vi "Autogenerate_Topology_Relation.vi"(5 "Goal District":string, 7 "Start District":string, 9 "PicAjust":T1={"TranslationVector"=[], "scale"=1.0, "Pitch（x) "=0.0, "Yaw（y)"=0.0, "Roll（z) "=0.0}, 10 "Cluster of 7 Type Data":T3(array[cluster])) -> (0 "District Name Array":string[](array[string]), 1 "Path Coodinate Array":dbl[][](array[numeric]), 2 "Path Relation topology":dbl[][](array[numeric]), 3 "Topology Matrix":dbl[][](array[numeric]), 4 "All Path Array":string[](array[string]), 8 "yidong":dbl[](array[numeric]))   [LabVIEW 2014]
doc: "通过数据生成各个房间、过道、楼梯的空间拓扑矩阵"
uses:
  <vilib>/Analysis/Matrix/Datatypes/RealMatrix.ctl
  <vilib>/Analysis/Matrix/NI_Matrix.lvlib
panel:
  in  "Scalar":dbl=0.06
  in  "Data Matrix":T2=[[0.0, 0.0, 0.0], [0.0, 11696.0, 0.0], [11414.5, 11843.9, 150.0], [14173.5, 5920.8, 150.0], [13501.3, 5521.4, 150.0]]
  in  "translation":cluster{"X":i32, "Y":i32}
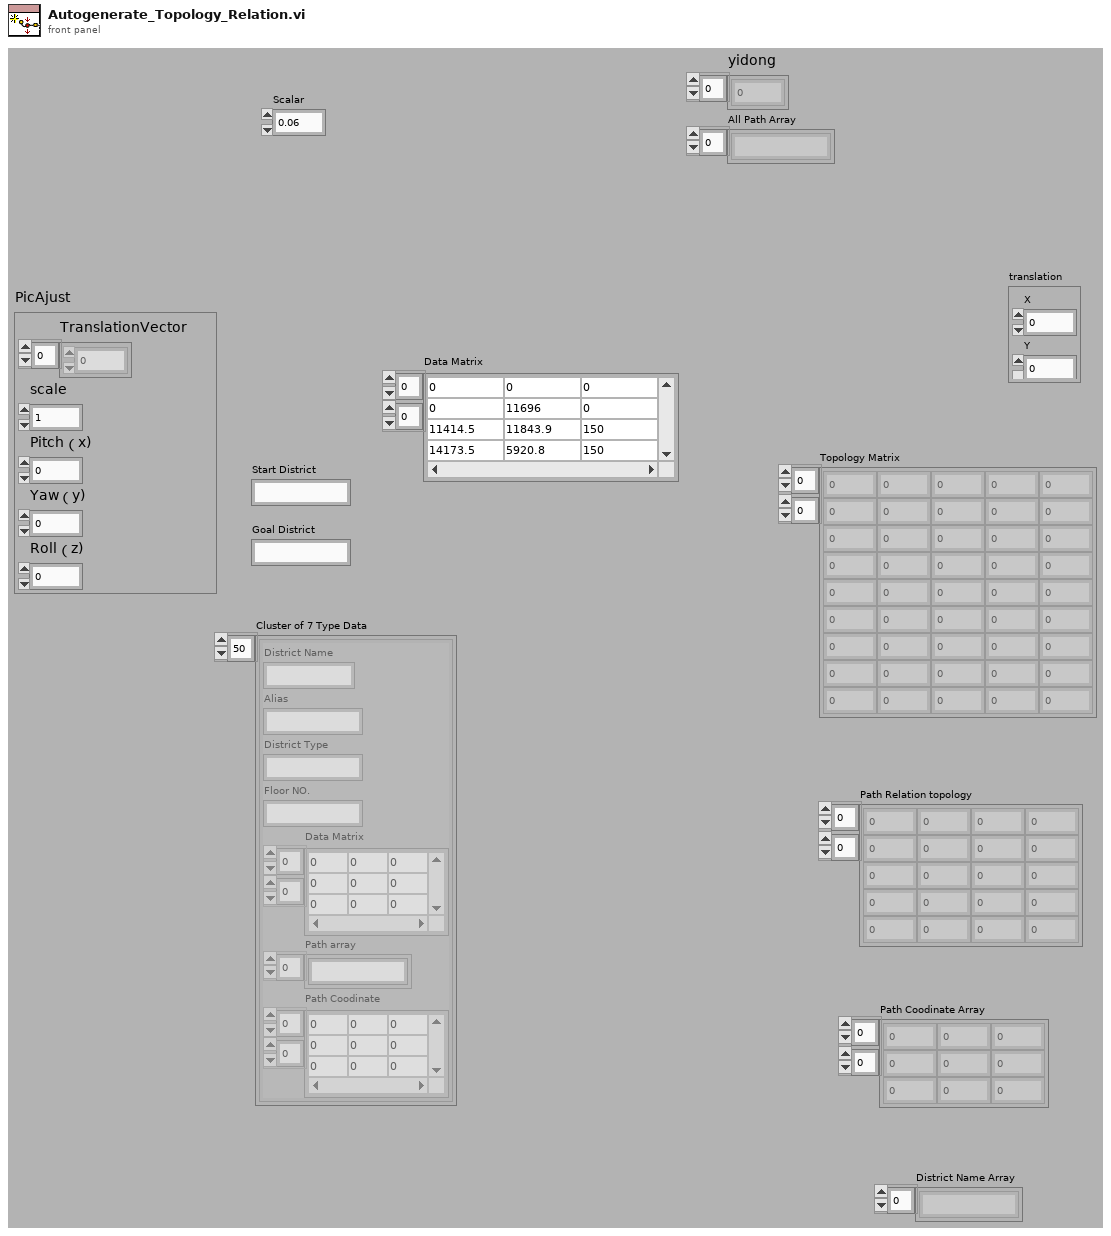
[diagram p1: front panel]
types:
  T1 = cluster{"TranslationVector":dbl[], "scale":dbl, "Pitch（x) ":dbl, "Yaw（y)":dbl, "Roll（z) ":dbl}
  T2 = typedef "NI_Matrix.lvlib/RealMatrix.ctl" = dbl[][]
  T3 = cluster{"District Name":string, "Alias":string, "District Type":string, "Floor NO.":string, "Data Matrix":T2, "Path array":string[], "Path Coodinate":T2}[]
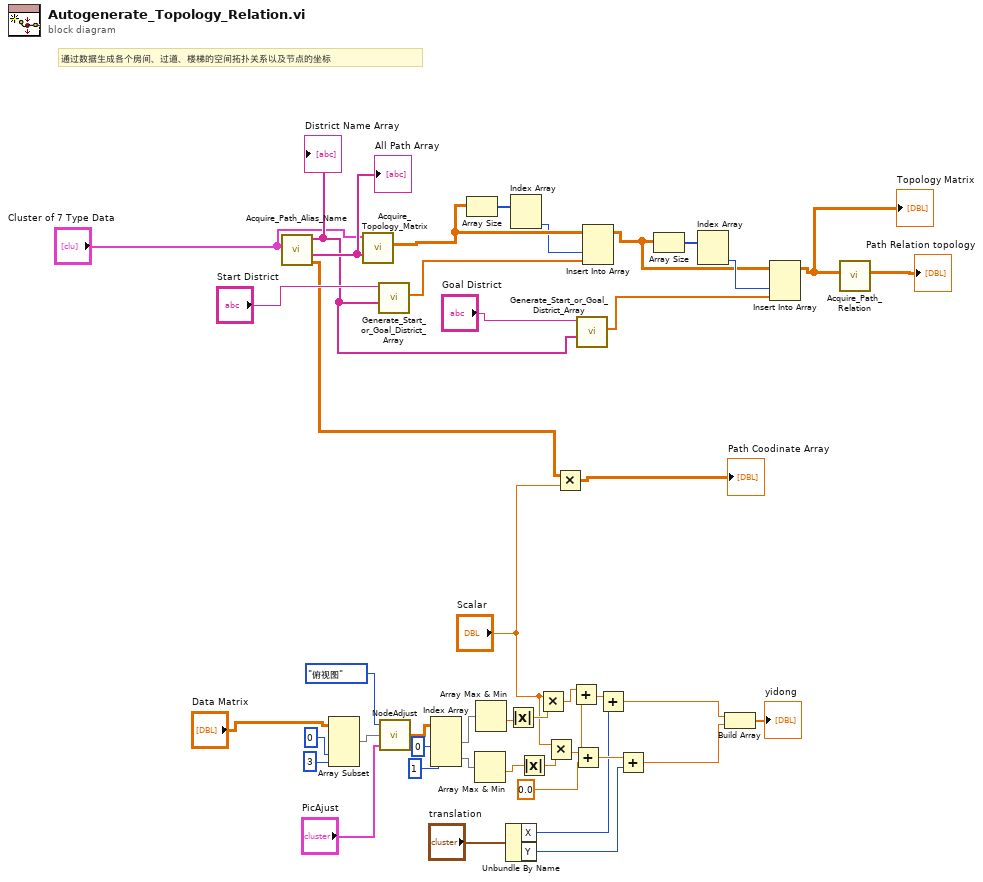
[diagram p0: block diagram]
diagram:
  w24 = 0.0 ("y")
  # "通过数据生成各个房间、过道、楼梯的空间拓扑关系以及节点的坐标"
  n1 = call "Acquire_Path_Alias_Name.vi"("Cluster of 7 Type Data"="Cluster of 7 Type Data") -> ("Path Coodinate Array"=w6:dbl[][], "All Path Array"=w44:string[], "District Name Array"=w31:string[])  [unwired: 7 in, 1 out]
  "District Name Array" <- w31
  "All Path Array" <- w44
  n2 = Array Subset(array="Data Matrix", index (col)=0 ("索引"), length (col)=3 ("长度")) -> (w16:T2)  [unwired: 2 in]
  n3 = call "Acquire_Topology_Matrix.vi"("All Path Array"=w44, "Cluster of 7 Type Data"="Cluster of 7 Type Data") -> ("Topology Matrix"=w42:dbl[][])  [unwired: 9 in]
  n4 = call "Generate_Start_or_Goal_District_Array .vi"("District Name Array"=w31, "Start_Goal District"="Start District") -> ("Compare District Array"=w39:dbl[])  [unwired: 9 in]
  n5 = call "NodeAdjust.vi"("PicAjust"="PicAjust", "NodeM"=w16, "视图"=enum16{"俯视图", "轴测图"}."俯视图" ("viewer")) -> ("NewNodeM"=w13:dbl[][])
  n6 = Index Array(array=w13, index (col) #1=0 ("禁用的索引 (列)"), index (col) #2=1 ("索引 (列)")) -> (element #1=w9:dbl[], element #2=w10:dbl[])  [unwired: 2 in]
  n7 = Array Size(array=w42) -> (size(s)=w41:i32[])
  n8 = Array Max & Min(array=w10) -> (min value=w22:dbl)  [unwired: 3 out]
  n9 = Array Max & Min ("数组最大值与最小值")(array=w9) -> (min value=w17:dbl)  [unwired: 3 out]
  n10 = Unbundle By Name("translation") -> ("X"=w27:i32, "Y"=w29:i32)
  n11 = Absolute Value(x=w17) -> (abs(x)=w18:dbl)
  n12 = Index Array(array=w41) -> (element #2=w40:i32)  [unwired: 2 in, 1 out]
  n13 = Absolute Value(x=w22) -> (abs(x)=w21:dbl)
  n14 = Multiply(x="Scalar", y=w18) -> (x*y=w19:dbl)
  n15 = Multiply(x="Scalar", y=w21) -> (x*y=w23:dbl)
  n16 = Multiply(x=w6, y="Scalar") -> (x*y=→"Path Coodinate Array":dbl[][])
  n17 = Add(x=w19, y=w24) -> (x+y=w26:dbl)
  n18 = Add(x=w23, y=w24) -> (x+y=w28:dbl)
  n19 = call "Generate_Start_or_Goal_District_Array .vi"("District Name Array"=w31, "Start_Goal District"="Goal District") -> ("Compare District Array"=w34:dbl[])  [unwired: 9 in]
  n20 = Insert Into Array(array=w42, index (col)=w40, new element=w39) -> (w35:dbl[][])  [unwired: 1 in]
  n21 = Add(x=w26, y=w27) -> (x+y=w3:dbl)
  n22 = Add(x=w28, y=w29) -> (x+y=w2:dbl)
  n23 = Array Size(array=w35) -> (size(s)=w36:i32[])
  n24 = Index Array(array=w36) -> (element #2=w37:i32)  [unwired: 2 in, 1 out]
  n25 = Build Array(w3, w2) -> (→"yidong":dbl[])
  n26 = Insert Into Array(array=w35, index (col)=w37, new element=w34) -> (w32:dbl[][])  [unwired: 1 in]
  "Topology Matrix" <- w32
  n27 = call "Acquire_Path_Relation.vi"("Topology Matrix"=w32) -> ("Path Relation topology"=→"Path Relation topology":dbl[][])  [unwired: 10 in]
